vi "10-Tap 8-Bit Camera with DRAM (Host).vi"() -> ()   [LabVIEW 2014]
doc: "This is the host VI for the 10-Tap 8-Bit Camera with DRAM example. This example demonstrates how to acquire images from a 10-tap, 8-bit, extended configuration, Camera Link camera and display the images on the host. This example supports area scan and line scan cameras for both continuous and finite acquisitions.\n\nThis example also demonstrates the use of DRAM as a frame buffer for very high speed acquisitions. Data packing and flow-control are also employed to maximize use of the available DRAM and FIFOs in terms of both memory space and performance.\n\nAdditionally, the example demonstrates the serial server, which allows third-party camera configuration utilities to communicate with the camera using the Camera Link serial interface while this VI is running."
uses:
  <vilib>/userdefined/High Color/nirio_resource_hc.ctl
  <vilib>/DAQmx/write.llb/DAQmx Write (Analog DBL 1Chan 1Samp).vi
  <vilib>/FPGAPlugInAG/PCIe-1473R/niLvFpga_Open_PCIe-1473R.vi
  <vilib>/rvi/interface/common/dynamic/niFpgaDynamicAddResources.vi
  <vilib>/FPGAPlugInAG/Dynamic/niLvFpga_Reset_Dynamic.vi
  <vilib>/Utility/error.llb/Error Cluster From Error Code.vi
  <vilib>/rvi/errors/niLvFpgaAdjustHostInterfaceError.vi
  <vilib>/FPGAPlugInAG/Dynamic/niLvFpga_Run_Dynamic.vi
  <vilib>/rvi/interface/common/niFpgaWaitOnOcc.vi
  <vilib>/FPGAPlugInAG/Dynamic/niLvFpga_Close_Dynamic.vi
  <vilib>/rvi/interface/nirviOpenFPGA/nirviOpenFPGA.xnode
  FPGA Bitfiles/10-Tap8-bitCamer_FPGATarget_10-Tap8-bitCamer_C490DC32.lvbitx
  10-Tap 8-Bit Camera with DRAM(FPGA).vi
  <vilib>/rvi/interface/nirviMethod/nirviMethod.xnode
  <vilib>/rvi/interface/nirviReadWriteControl/nirviReadWriteControl.xnode
  <vilib>/rvi/interface/nirviCloseFPGA/nirviCloseFPGA.xnode
  <vilib>/rvi/interface/Simulation/niFpgaSimulationCallBeginRW.vi
  <vilib>/rvi/errors/niLvFpgaMergeErrorWithErrorCode.vi
  NiFpgaLv.dll
  <vilib>/FPGAPlugInAG/Dynamic/niLvFpga_ConfigureFifo_Dynamic.vi
  <vilib>/FPGAPlugInAG/Dynamic/niLvFpga_StartFifo_Dynamic.vi
  <vilib>/FPGAPlugInAG/Dynamic/niLvFpga_ReadFifo_Dynamic.vi
  <vilib>/vision/NI_Vision_Development_Module.lvlib
panel:
  out "YofFishHead":sgl
  out "XofFishHead":dbl
  in  "Ly":sgl=30.0
  in  "Lx":dbl=50.0
  out "TimeDelay":dbl
  out "RegionSelected":T1(plugin-control)
  in  "Threshold":u8=96
  out "Objects":T2(array[cluster]) {"Aspect Ratio" format="%.2f"; "Orientation" format="%.2f"; "Area" format="%.2f"; "Object Center"."Y" format="%.2f"; "Object Center"."X" format="%.2f"}
  in  "Machine Vision Settings":T3={"Objects"=0, "Threshold"=128, "Reject Border"=FALSE, "Fill Holes"=FALSE, "Min Object Size"=TRUE, "Min Size"=10000, "Max Object Size"=FALSE, "Max Size"=100, "Show Search Area"=FALSE, "Show Center"=TRUE, "Show Bounding Box"=TRUE} {"Objects" items=["Bright Objects", "Dark Objects"]; "Threshold" min=1 max=999999999 step=1; "Max Size" min=1 max=999999999 step=1; "Min Size" min=1 max=999999999 step=1}
  in  "长度2_LeftToRight":i32=300
  in  "索引2_LeftEdge":i32=250
  in  "长度1_UpToLow":i32=400
  in  "索引1_UpEdge":i32=290
  out "image":u8[][](array[numeric])
  in  "SpeedFactor":dbl=1.0
  in  "Offset":dbl=150.0
  in  "Y_Target":dbl=384.0
  in  "X_Target":dbl=520.0
  in  "Y_LowEdge_ofCenter":fxp<+,32,16>=440.0 format="%#_21g"
  in  "X_RightEdge_ofCenter":fxp<+,32,16>=600.0 format="%#_21g"
  in  "Y_HighEdge_ofCenter":fxp<+,32,16>=270.0 format="%#_21g"
  in  "X_LeftEdge_ofCenter":fxp<+,32,16>=440.0 format="%#_21g"
  out "Y_edge":u16[](array[numeric])
  out "X_edge":u16[](array[numeric])
  out "Centroid":fxp<+,32,16>[](array[numeric])
  in  "DMA Buffer Size\n(In Images)":u32=64 caption="DMA Buffer Size"
  in  "Signal Mapping":T4(ring)=enum."Basler 10-tap"
  out "Acq In Progress":bool
  in  "Line Scan":bool
  in  "Frames To Acquire":u32 caption="Frames To Acquire\n(0 = infinite)"
  in  "Cancel":bool
  out "Acq'd Frame Width":u32
  in  "Stopped":bool
  in  "RIO Device":T5="Horizontal"
  out "DMA Write Timeout":bool
  in  "Start Serial Server":bool=TRUE
  out "Frames Acq'd":u32
  out "Acq'd Frame Height":u32
  out "Image":T1(plugin-control)
  in  "Acquire":bool
  in  "Stop":bool
  in  "Image Height":u32=768 max=65535
  in  "Image Width":u32=1040 max=65535 step=40
  out "Initialized":bool
  # "对鱼的不同方位进行不同的微调。"
  # "右边四个参数是一个\n长方形框的四个边，\n只有当FPGA计算出来\n的中心在这个框内的\n时候才会使用PC进行\n处理。"
  # "右边四个参数也是\n一个长方形的框，\n他是PC进行处理的\n范围，它的大小直\n接影响PC处理的速\n度。"
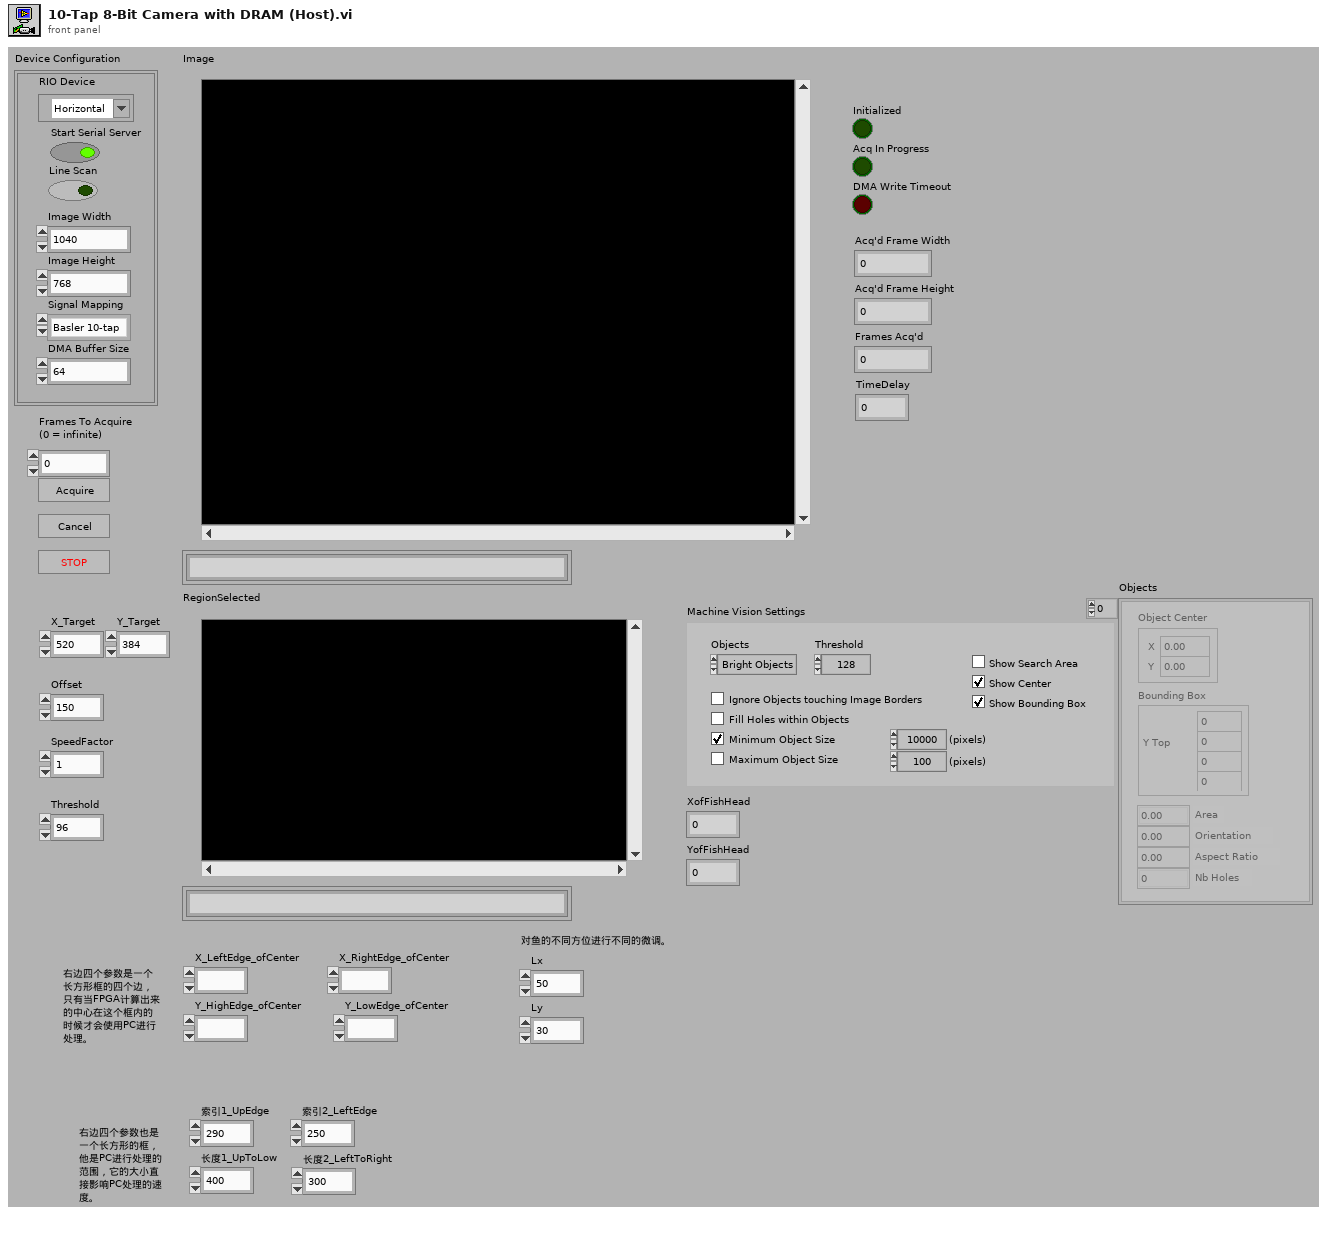
[diagram p1: front panel]
types:
  T1 = typedef "IMAQ Image.ctl" = refnum<image>
  T2 = cluster{"Object Center":cluster{"X":sgl, "Y":sgl}, "Bounding Box":cluster{"X Left":i32, "Y Top":i32, "X Right":i32, "Y Bottom":i32}, "Area":sgl, "Orientation":sgl, "Aspect Ratio":sgl, "Nb Holes":i32}[]
  T3 = cluster{"Objects":u16, "Threshold":i32, "Reject Border":bool, "Fill Holes":bool, "Min Object Size":bool, "Min Size":i32, "Max Object Size":bool, "Max Size":i32, "Show Search Area":bool, "Show Center":bool, "Show Bounding Box":bool}
  T4 = enum8{"Standard", "Basler 10-tap", "Vosskühler 10-tap"}
  T5 = typedef "nirio_resource_hc.ctl" = tag
  T6 = typedef "Image Type" = u32
  T7 = enum16{"big-endian, network order", "native, host order", "little-endian"}
  T8 = enum32{"AutoM", "Close", "Dilate", "Erode", "Gradient", "Gradient out", "Gradient in", "Hit miss", "Open", "PClose", "POpen", "Thick", "Thin"}
  T9 = cluster{"Object Center":cluster{"X":sgl, "Y":sgl}, "Bounding Box":cluster{"X Left":i32, "Y Top":i32, "X Right":i32, "Y Bottom":i32}, "Area":sgl, "Orientation":sgl, "Aspect Ratio":sgl, "Nb Holes":i32}
  T10 = cluster{"X Left":i32, "Y Top":i32, "X Right":i32, "Y Bottom":i32}
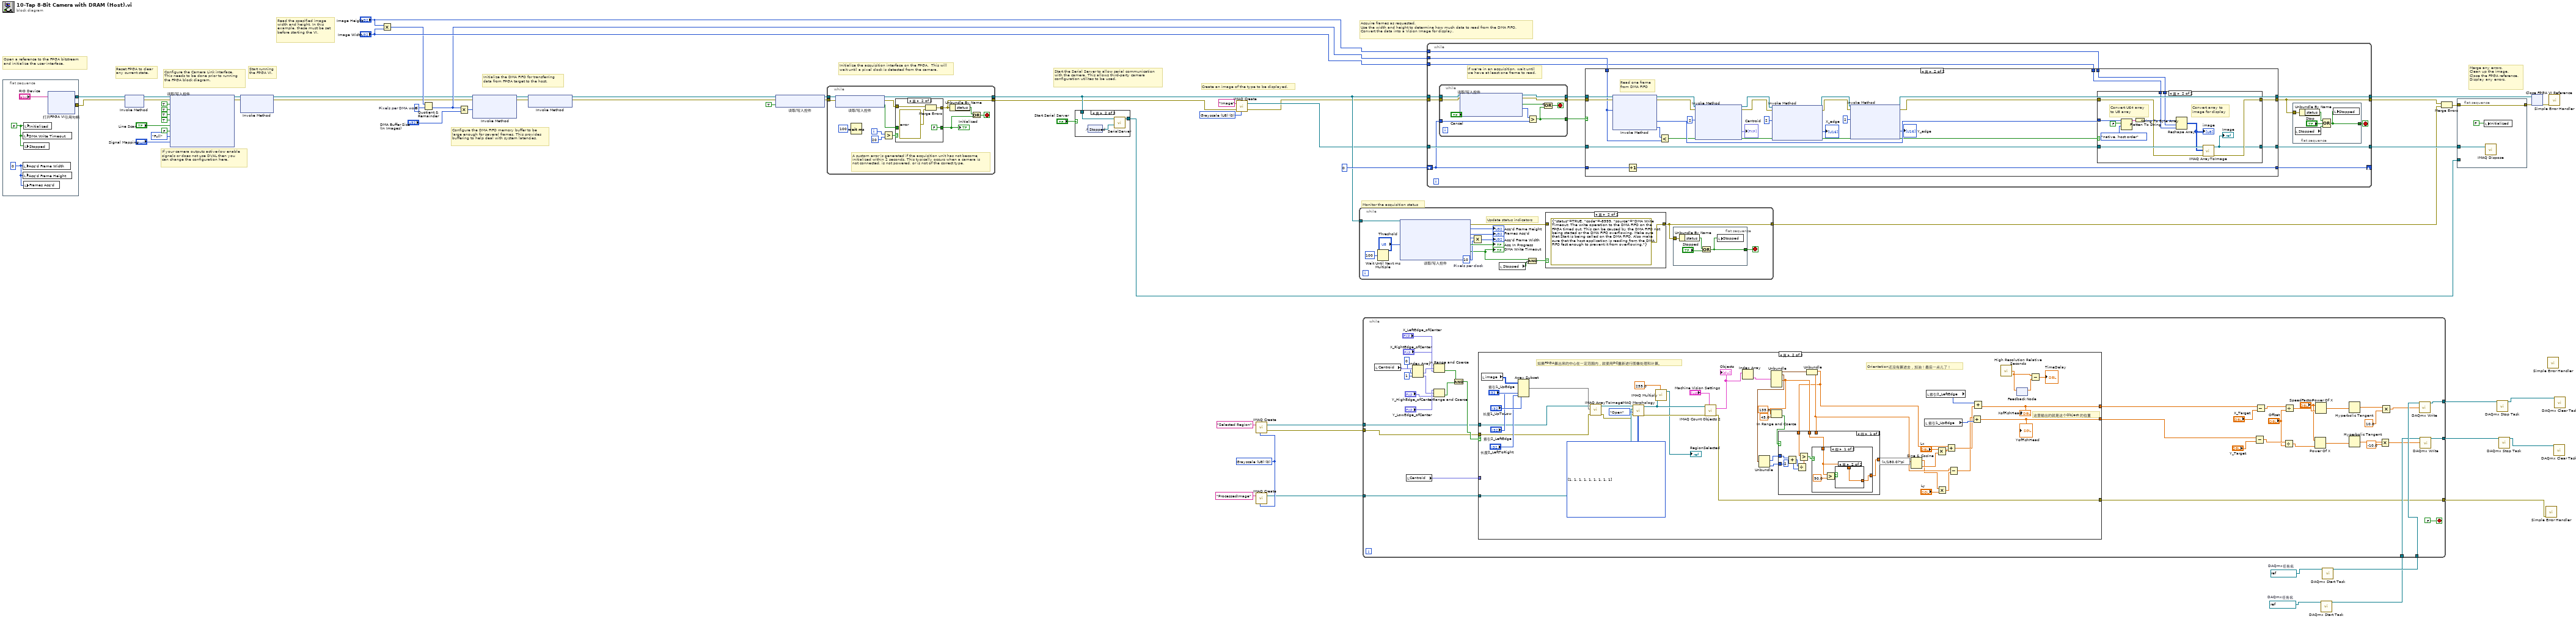
[diagram p0: block diagram]
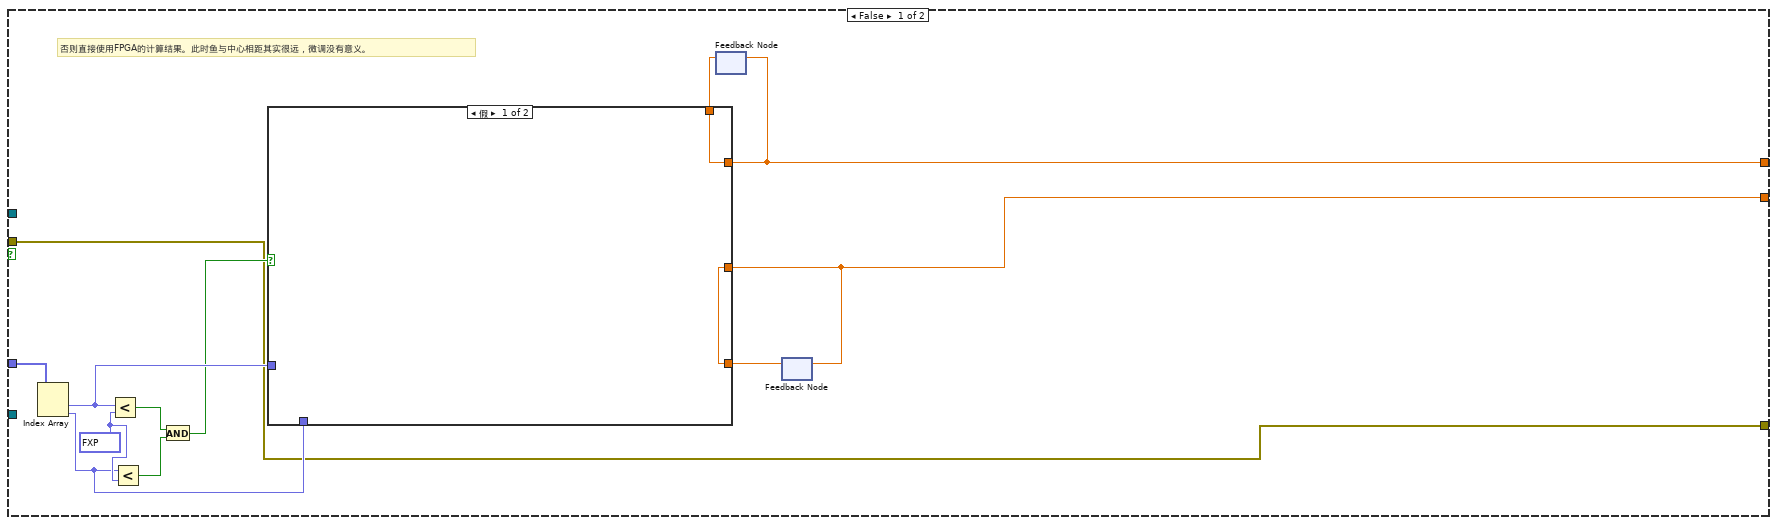
[diagram p2: hidden frame]
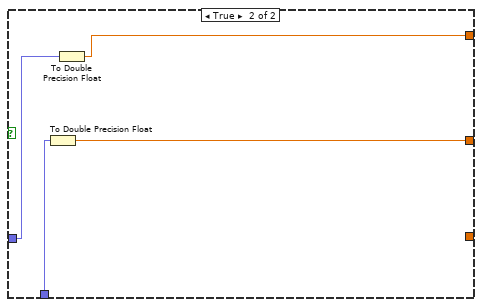
[diagram p3: hidden frame]
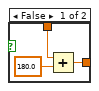
[diagram p4: hidden frame]
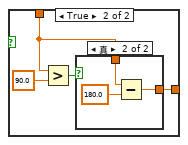
[diagram p5: hidden frame]
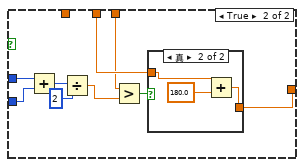
[diagram p7: hidden frame]
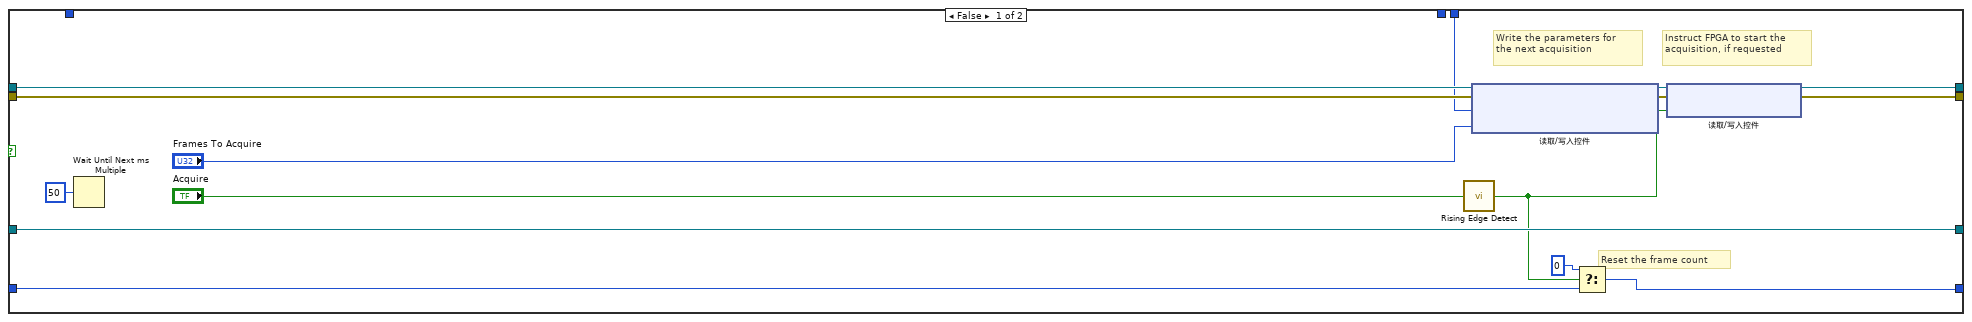
[diagram p11: hidden frame]
diagram:
  w4 = T6 0 items=["Grayscale (U8)", "Grayscale (I16)", "Grayscale (SGL)", "Complex (CSG)", "RGB (U32)", "HSL (U32)", "RGB (U64)", "Grayscale (U16)"] ("Image Type")
  w12 = refnum<k21> "Stage_Y"  # DAQmx任务名
  w15 = refnum<k21> "Stage_X"  # DAQmx任务名
  w21 = u32 8  # Pixels per DMA word
  w57 = T6 0 items=["Grayscale (U8)", "Grayscale (I16)", "Grayscale (SGL)", "Complex (CSG)", "RGB (U32)", "HSL (U32)", "RGB (U64)", "Grayscale (U16)"] ("Image Type")
  # "If your camera outputs active-low enable\nsignals or does not use DVAL then you \ncan change the configuration here."
  # "Configure the DMA FIFO memory buffer to be\nlarge enough for several frames. This provides\nbuffering to help deal with system latencies."
  # "Start running\nthe FPGA VI."
  # "Reset FPGA to clear\nany current state."
  # "Read the specified image\nwidth and height. In this\nexample, these must be set\nbefore starting the VI."
  # "Merge any errors.\nClean up the image.\nClose the FPGA reference.\nDisplay any errors."
  # "Acquire frames as requested.\nUse the width and height to determine how much data to read from the DMA FIFO.\nConvert the data into a Vision Image for display."
  # "Monitor the acquisition status"
  # "Start the Serial Server to allow serial communication\nwith the camera. This allows third-party camera\nconfiguration utilites to be used."
  # "Create an image of the type to be displayed."
  # "Initialize the acquisition interface on the FPGA.  This will\nwait until a pixel clock is detected from the camera."
  # "Initialize the DMA FIFO for transferring\ndata from FPGA target to the host."
  # "Configure the Camera Link interface.\nThis needs to be done prior to running\nthe FPGA block diagram."
  # "Open a reference to the FPGA bitstream\nand initialize the user interface."
  n1 = flat-sequence {
    tunnel: [w63] -> w48
    tunnel: [w62] -> w61
    frame #0 {
      w66 = u32 0 ("Num Lines Acq'd")
      w65 = FALSE ("stop")
      n2 = local write "DMA Write Timeout"(w65) -> ()
      n3 = local write "Acq'd Frame Width"(w66) -> ()
      n4 = local write "Acq'd Frame Height"(w66) -> ()
      n5 = local write "Stopped"(w65) -> ()
      n6 = local write "Frames Acq'd"(w66) -> ()
      n7 = local write "Initialized"(w65) -> ()
      n8 = xnode "打开FPGA VI引用句柄"("资源名称"="RIO Device") -> ("FPGA VI引用输出"=w63:refnum<k20>, "错误输出"=w62:errorcluster)  [unwired: 1 in]
    }
  }
  n9 = xnode "Invoke Method"("FPGA VI引用输入"=w48, "错误输入"=w61) -> ("FPGA VI引用输出"=w38:refnum<k20>, "错误输出"=w41:errorcluster)
  n10 = xnode "读取/写入控件"("FPGA VI引用输入"=w38, "错误输入"=w41, "CL Config.FVAL Active High"=TRUE ("IO Module Config.CL FVAL Active High"), "CL Config.LVAL Active High"=TRUE ("IO Module Config.CL LVAL Active High"), "CL Config.DVAL Active High"=TRUE ("IO Module Config.CL DVAL Active High"), "CL Config.Spare Active High"=TRUE ("IO Module Config.CL Spare Active High"), "CL Config.Line Scan"="Line Scan", "Acq Control.Ignore DVAL"=FALSE ("CL Config.Line Scan"), "CL Config.Configuration"=enum8{"Base", "Medium", "Full"}."Full", "CL Config.Signal Mapping"="Signal Mapping") -> ("FPGA VI引用输出"=w42:refnum<k20>, "错误输出"=w40:errorcluster)
  n11 = xnode "Invoke Method"("FPGA VI引用输入"=w42, "错误输入"=w40) -> ("FPGA VI引用输出"=w18:refnum<k20>, "错误输出"=w17:errorcluster)  [unwired: 1 in]
  n12 = Multiply(x="Image Height", y="Image Width") -> (x*y=w20:u32)
  n13 = Quotient & Remainder(x=w20, y=w21) -> (floor(x/y)=w19:u32)  [unwired: 1 out]
  n14 = Multiply(x=w19, y="DMA Buffer Size\n(In Images)") -> (x*y=w32:u32)
  n15 = xnode "Invoke Method"("FPGA VI引用输入"=w18, "错误输入"=w17, "请求的深度"=w32) -> ("FPGA VI引用输出"=w16:refnum<k20>, "错误输出"=w47:errorcluster)  [unwired: 1 out]
  n16 = xnode "Invoke Method"("FPGA VI引用输入"=w16, "错误输入"=w47) -> ("FPGA VI引用输出"=w33:refnum<k20>, "错误输出"=w46:errorcluster)
  n17 = xnode "读取/写入控件"("FPGA VI引用输入"=w33, "错误输入"=w46, "Acq Control.Initialize"=TRUE ("Arm Acquisition")) -> ("FPGA VI引用输出"=w60:refnum<k20>, "错误输出"=w59:errorcluster)
  n18 = while {
    tunnel: w60 -> [w74]
    tunnel: w59 -> [w73]
    tunnel: [w72] -> w29
    tunnel: [w76] -> w28
    i -> [w68]
    stop <- w79 stop-if-true
    # "A custom error is generated if the acquisition unit has not become\ninitialized within 2 seconds. This typically occurs when a camera is\nnot connected, is not powered, or is not of the correct type."
    n19 = xnode "读取/写入控件"("FPGA VI引用输入"=w74, "错误输入"=w73) -> ("FPGA VI引用输出"=w72:refnum<k20>, "错误输出"=w71:errorcluster, "Acq Status.Initialized"=w70:bool)
    n20 = Wait (ms)(milliseconds to wait=u32 100) -> ()  [unwired: 1 out]
    n21 = Greater?(x=w68, y=20) -> (0:w69:bool)
    n22 = case shown="真" w69 {
      tunnel: [w81 FALSE] -> w75
      tunnel: w70 -> [w81 _]
      tunnel: w71 -> [w80 w83]
      tunnel: [w80 w85] -> w76
      frame False {
      }
      frame True {
        n23 = Merge Errors(w83, errorcluster {"status"=TRUE, "code"=-8999, "source"="Acquisition Initialization: This error typically occurs when a camera is not properly connected, is not powered, or is not of the correct type."} ("error in")) -> (w85:errorcluster)
      }
    }
    "Initialized" <- w75
    n24 = Unbundle By Name(w76) -> ("status"=w78:bool)
    n25 = Or(x=w78, y=w75) -> (x .or. y?=w79:bool)
  }
  n26 = case shown="真" "Start Serial Server" {
    tunnel: [_ w86] -> w49
    tunnel: w29 -> [_ w87]
    frame False {
    }
    frame True {
      n27 = control-ref of="Stopped"() -> (w88:refnum<vi>)
      n28 = call "SerialServer.vi"("Stop Refnum"=w88, "FPGA VI Reference In"=w87) -> ("FPGA VI Reference Out"=w86:refnum<k20>)  [unwired: 5 in]
    }
  }
  n29 = call "IMAQ Create"("Image Name"="Image", "Image Type"=w57, "error in (no error)"=w28) -> ("New Image"=w25:T1, "error out"=w24:errorcluster)  [unwired: 2 in]
  n30 = call "IMAQ Create"("Image Name"="Selected Region", "Image Type"=w4) -> ("New Image"=w6:T1, "error out"=w5:errorcluster)  [unwired: 3 in]
  n31 = call "IMAQ Create"("Image Name"="ProcessedImage", "Image Type"=w4) -> ("New Image"=w2:T1)  [unwired: 3 in, 1 out]
  n32 = while {
    tunnel: w29 -> [w100]
    tunnel: [w103] -> w43
    stop <- w102 stop-if-true
    w93 = u32 10  # Pixels per clock
    # "Update status indicators"
    n33 = Wait Until Next ms Multiple(millisecond multiple=u32 100) -> ()  [unwired: 1 out]
    n34 = xnode "读取/写入控件"("FPGA VI引用输入"=w100, "Threshold"="Threshold") -> ("错误输出"=w99:errorcluster, "Acq Status.Lines Per Frame"=→"Acq'd Frame Height":u32, "Acq Status.Frames Acq'd"=→"Frames Acq'd":u32, "Acq Status.Clocks Per Line"=w94:u32, "Acq Status.Acq In Progress"=→"Acq In Progress":bool, "Acq Status.DMA Write Timeout"=w91:bool)  [unwired: 1 in, 1 out]
    "DMA Write Timeout" <- w91
    n35 = Multiply(x=w94, y=w93) -> (x*y=→"Acq'd Frame Width":u32)
    n36 = local read "Stopped"() -> (w90:bool)
    n37 = Compound Arithmetic op=AND(w91, invert w90) -> (w92:bool)
    n38 = case shown="真" w92 {
      tunnel: w99 -> [w108 _]
      tunnel: [w108 errorcluster {"status"=TRUE, "code"=-8999, "source"="DMA Write Timeout: The write operation to the DMA FIFO on the FPGA timed out. This can be caused by the DMA FIFO not being started or the DMA FIFO overflowing. Make sure that Start is being called on the DMA FIFO. Also make sure that the host application is reading from the DMA FIFO fast enough to prevent it from overflowing."} ("error out")] -> w103
      frame False {
      }
      frame True {
      }
    }
    n39 = flat-sequence {
      tunnel: w103 -> [w107]
      tunnel: [w105] -> w102
      frame #0 {
        n40 = Unbundle By Name(w107) -> ("status"=w106:bool)
        n41 = Or(x=w106, y="Stopped") -> (x .or. y?=w105:bool)
        n42 = local write "Stopped"(w105) -> ()
      }
    }
  }
  n43 = while {
    tunnel: w29 -> [w116]
    tunnel: w24 -> [w115]
    tunnel: w19 -> [w124]
    tunnel: "Image Height" -> [w123]
    tunnel: "Image Width" -> [w122]
    tunnel: w25 -> [w121]
    tunnel: [w119] -> w44
    tunnel: [w120] -> w56
    tunnel: [w117] -> w51
    shift-right: [w111] -> _
    shift-left: u32 0 -> [w110]
    stop <- w118 stop-if-true
    # "If we're in an acquisition, wait until\nwe have at least one frame to read."
    n44 = while {
      tunnel: w116 -> [w131]
      tunnel: w115 -> [w130]
      tunnel: [w128] -> w114
      tunnel: [w129] -> w113
      tunnel: w110 -> [w134]
      tunnel: [w132] -> w112
      stop <- w133 stop-if-true
      n45 = xnode "读取/写入控件"("FPGA VI引用输入"=w131, "错误输入"=w130, "Acq Control.Cancel Acq"="Cancel") -> ("FPGA VI引用输出"=w129:refnum<k20>, "错误输出"=w128:errorcluster, "Acq Status.Acq In Progress"=w127:bool, "Acq Status.Frames Acq'd"=w126:u32)
      n46 = Greater?(x=w126, y=w134) -> (0:w132:bool)
      n47 = Compound Arithmetic op=OR(invert w127, w132) -> (w133:bool)
    }
    n48 = case shown="真" w112 {
      tunnel: w113 -> [w150 w176]
      tunnel: w114 -> [w149 w175]
      tunnel: w124 -> [_ w169]
      tunnel: w123 -> [w143 w181]
      tunnel: w122 -> [_ w180]
      tunnel: w121 -> [w154 w179]
      tunnel: [w145 w178] -> w119
      tunnel: [w148 w162] -> w120
      tunnel: [w154 w177] -> w117
      tunnel: w110 -> [w151 w174]
      tunnel: [w153 w173] -> w111
      frame False {
        # "Reset the frame count"
        # "Instruct FPGA to start the\nacquisition, if requested"
        # "Write the parameters for\nthe next acquisition"
        n49 = Wait Until Next ms Multiple(millisecond multiple=u32 50) -> ()  [unwired: 1 out]
        n50 = call "Rising Edge Detect.vi"("Input"="Acquire") -> ("Pulse"=w140:bool)  [unwired: 4 in]
        n51 = xnode "读取/写入控件"("FPGA VI引用输入"=w150, "错误输入"=w149, "Acq Control.Line Scan Height"=w143, "Acq Control.Frames To Acq"="Frames To Acquire") -> ("FPGA VI引用输出"=w147:refnum<k20>, "错误输出"=w146:errorcluster)
        n52 = Select(t=u32 0, s=w140, f=w151) -> (s? t:f=w153:u32)
        n53 = xnode "读取/写入控件"("FPGA VI引用输入"=w147, "错误输入"=w146, "Acq Control.Acquire"=w140) -> ("FPGA VI引用输出"=w148:refnum<k20>, "错误输出"=w145:errorcluster)
      }
      frame True {
        # "Read one frame\nfrom DMA FIFO"
        n54 = xnode "Invoke Method"("FPGA VI引用输入"=w176, "错误输入"=w175, "元素数量"=w169) -> ("FPGA VI引用输出"=w168:refnum<k20>, "错误输出"=w167:errorcluster, "数据"=w172:u64[], "剩余元素"=w170:u32)  [unwired: 1 in]
        n55 = Increment(x=w174) -> (x+1=w173:u32)
        n56 = Less?(x=w170, y=w169) -> (x < y?=w171:bool)
        n57 = xnode "Invoke Method"("FPGA VI引用输入"=w168, "错误输入"=w167, "元素数量"=u32 2) -> ("FPGA VI引用输出"=w165:refnum<k20>, "错误输出"=w164:errorcluster, "数据"=→"Centroid":fxp<+,32,16>[])  [unwired: 1 in, 1 out]
        n58 = xnode "Invoke Method"("FPGA VI引用输入"=w165, "错误输入"=w164, "元素数量"=u32 2) -> ("FPGA VI引用输出"=w163:refnum<k20>, "错误输出"=w161:errorcluster, "数据"=→"X_edge":u16[])  [unwired: 1 in, 1 out]
        n59 = xnode "Invoke Method"("FPGA VI引用输入"=w163, "错误输入"=w161, "元素数量"=u32 2) -> ("FPGA VI引用输出"=w162:refnum<k20>, "错误输出"=w160:errorcluster, "数据"=→"Y_edge":u16[])  [unwired: 1 in, 1 out]
        n60 = case shown="真" w171 {
          tunnel: w181 -> [_ w195]
          tunnel: w180 -> [_ w194]
          tunnel: w179 -> [w183 w193]
          tunnel: w160 -> [w182 w192]
          tunnel: [w182 w191] -> w178
          tunnel: [w183 w190] -> w177
          tunnel: w172 -> [_ w187]
          frame False {
            # "Do not display the image if we're falling behind in the acquisition."
          }
          frame True {
            # "Convert U64 array\nto U8 array"
            # "Convert array to\nimage for display"
            n61 = Flatten To String(anything=w187, prepend array or string size? (T)=FALSE, byte order (0:big-endian, network order)=T7."native, host order") -> (data string=w185:string)  [unwired: 1 in, 2 out]
            n62 = String To Byte Array(string=w185) -> (unsigned byte array=w184:u8[])
            n63 = Reshape Array(w184, w195, w194) -> (w189:u8[][])
            "image" <- w189
            n64 = call "IMAQ ArrayToImage"("error in (no error)"=w192, "Image Pixels (U8)"=w189, "Image"=w193) -> ("error out"=w191:errorcluster, "Image Out"=w190:T1)  [unwired: 7 in]
            "Image" <- w190
          }
        }
      }
    }
    n65 = flat-sequence {
      tunnel: w119 -> [w137]
      tunnel: [w136] -> w118
      frame #0 {
        n66 = local read "Stopped"() -> (w135:bool)
        n67 = Unbundle By Name(w137) -> ("status"=w138:bool)
        n68 = Compound Arithmetic op=OR(w138, "Stop", w135) -> (w136:bool)
        n69 = local write "Stopped"(w136) -> ()
      }
    }
  }
  n70 = call <vilib>:"DAQmx Start Task.vi"("task/channels in"=w12) -> ("task out"=w13:refnum<k21>)  [unwired: 13 in, 1 out]
  n71 = call <vilib>:"DAQmx Start Task.vi"("task/channels in"=w15) -> ("task out"=w14:refnum<k21>)  [unwired: 13 in, 1 out]
  n72 = while {
    tunnel: w14 -> [w228]
    tunnel: w13 -> [w227]
    tunnel: [w226] -> w11
    tunnel: [w225] -> w10
    tunnel: w6 -> [w206]
    tunnel: w5 -> [w205]
    tunnel: w2 -> [w204]
    tunnel: [w202] -> w1
    stop <- FALSE stop-if-true
    n73 = local read "Centroid"() -> (w235:fxp<+,32,16>[])
    n74 = local read "Centroid"() -> (w224:fxp<+,32,16>[])
    n75 = Index Array(array=w235, index #1=0 ("索引"), index #2=1 ("索引")) -> (element #1=w234:fxp<+,32,16>, element #2=w231:fxp<+,32,16>)
    n76 = In Range and Coerce(upper limit="Y_LowEdge_ofCenter", x=w231, lower limit="Y_HighEdge_ofCenter") -> (In Range?=w229:bool)  [unwired: 1 out]
    n77 = In Range and Coerce(upper limit="X_RightEdge_ofCenter", x=w234, lower limit="X_LeftEdge_ofCenter") -> (In Range?=w230:bool)  [unwired: 1 out]
    n78 = And(x=w230, y=w229) -> (x .and. y?=w207:bool)
    n79 = case shown="真" w207 {
      tunnel: w224 -> [w247 _]
      tunnel: [w240 w283] -> w221
      tunnel: [w238 w281] -> w219
      tunnel: w206 -> [_ w295]
      tunnel: w205 -> [w236 w294]
      tunnel: w204 -> [_ w291]
      tunnel: [w236 w284] -> w202
      frame False {
        w246 = fxp<+,32,16> 10000.0 ("y")
        # "否则直接使用FPGA的计算结果。此时鱼与中心相距其实很远，微调没有意义。"
        n80 = Index Array(array=w247) -> (element #1=w243:fxp<+,32,16>, element #2=w242:fxp<+,32,16>)  [unwired: 2 in]
        n81 = Less?(x=w243, y=w246) -> (x < y?=w245:bool)
        n82 = Less?(x=w242, y=w246) -> (x < y?=w244:bool)
        n83 = And(x=w245, y=w244) -> (x .and. y?=w241:bool)
        n84 = feedback #1() -> (w239:dbl)  [unwired: 1 in]
        n85 = feedback #2() -> (w237:dbl)  [unwired: 1 in]
        n86 = case shown="假" w241 {
          tunnel: w243 -> [_ w253]
          tunnel: w242 -> [_ w252]
          tunnel: [w249 w251] -> w240
          tunnel: [w248 w250] -> w238
          tunnel: w239 -> [w249 _]
          tunnel: w237 -> [w248 _]
          frame False {
          }
          frame True {
            n87 = To Double Precision Float(number=w252) -> (double precision float=w250:dbl)
            n88 = To Double Precision Float(number=w253) -> (double precision float=w251:dbl)
          }
        }
        n89 = feedback-in #1(w240) -> ()
        n90 = feedback-in #2(w238) -> ()
      }
      frame True {
        # "如果FPGA算出来的中心在一定范围内，就使用PC重新进行图像处理和计算。"
        # "Orientation还没有算进去，加油！最后一点儿了！"
        # "这里输出的就是这个Object 的位置"
        n91 = local read "image"() -> (w301:u8[][])
        n92 = Array Subset(array=w301, index (row)="索引1_UpEdge", length (row)="长度1_UpToLow", index (col)="索引2_LeftEdge", length (col)="长度2_LeftToRight") -> (w296:u8[][])
        n93 = call "IMAQ ArrayToImage"("error in (no error)"=w294, "Image Pixels (U8)"=w296, "Image"=w295) -> ("error out"=w290:errorcluster, "Image Out"=w292:T1)  [unwired: 7 in]
        n94 = call "IMAQ Morphology"("Structuring Element"=i32[][] [[1, 1, 1], [1, 1, 1], [1, 1, 1]], "error in (no error)"=w290, "Operation"=T8."Open", "Image Dst"=w291, "Image Src"=w292) -> ("error out"=w289:errorcluster, "Image Dst Out"=w279:T1)  [unwired: 5 in]
        n95 = call "IMAQ Multiply"("Image Src A"=w279, "Constant"=255.0) -> ("Image Dst Out"=→"RegionSelected":T1)  [unwired: 5 in, 1 out]
        n96 = call "IMAQ Count Objects 2"("Settings"="Machine Vision Settings", "error in (no error)"=w289, "Image"=w279) -> ("error out"=w284:errorcluster, "Objects"=w276:T2)  [unwired: 4 in, 3 out]
        "Objects" <- w276
        n97 = Index Array(array=w276) -> (element=w286:T9)  [unwired: 1 in]
        n98 = Unbundle(w286) -> ("Object Center"=w285:cluster{"X":sgl, "Y":sgl}, "Bounding Box"=w272:T10, "Orientation"=w258:sgl)  [unwired: 3 out]
        n99 = Unbundle(w272) -> ("Y Top"=w271:i32, "Y Bottom"=w270:i32)  [unwired: 2 out]
        n100 = In Range and Coerce(upper limit=sgl 135.0 ("上限"), x=w258, lower limit=sgl 45.0 ("下限")) -> (In Range?=w255:bool)  [unwired: 1 out]
        n101 = Unbundle(w285) -> ("X"=w254:sgl, "Y"=w263:sgl)
        n102 = case shown="假" w255 {
          tunnel: w271 -> [w310 w332]
          tunnel: w270 -> [w309 w331]
          tunnel: w258 -> [w303 w329]
          tunnel: [w302 w328] -> w267
          tunnel: w263 -> [_ w327]
          tunnel: w254 -> [w307 _]
          frame False {
            n103 = Add(x=w310, y=w309) -> (x+y=w308:i32)
            n104 = Divide(x=w308, y=2) -> (x/y=w305:dbl)
            n105 = Greater?(x=w307, y=w305) -> (0:w306:bool)
            n106 = case shown="假" w306 {
              tunnel: w303 -> [w312 w320]
              tunnel: [w311 w319] -> w302
              frame False {
                n107 = Greater?(x=w312, y=90.0) -> (0:w313:bool)
                n108 = case shown="真" w313 {
                  tunnel: w312 -> [w316 w318]
                  tunnel: [w315 w318] -> w311
                  frame False {
                    n109 = Add(x=w316, y=180.0) -> (x+y=w315:dbl)
                  }
                  frame True {
                  }
                }
              }
              frame True {
                n110 = Greater?(x=w320, y=90.0) -> (0:w321:bool)
                n111 = case shown="真" w321 {
                  tunnel: w320 -> [w323 w325]
                  tunnel: [w323 w324] -> w319
                  frame False {
                  }
                  frame True {
                    n112 = Subtract(x=w325, y=180.0) -> (x-y=w324:dbl)
                  }
                }
              }
            }
          }
          frame True {
            n113 = Add(x=w332, y=w331) -> (x+y=w335:i32)
            n114 = Divide(x=w335, y=2) -> (x/y=w333:dbl)
            n115 = Greater?(x=w327, y=w333) -> (0:w330:bool)
            n116 = case shown="真" w330 {
              tunnel: w329 -> [w336 w339]
              tunnel: [w336 w337] -> w328
              frame False {
              }
              frame True {
                n117 = Add(x=w339, y=sgl 180.0) -> (x+y=w337:sgl)
              }
            }
          }
        }
        n118 = expression code="(x/180.0)*pi" ("degrees to radians")(w267) -> (w266:dbl)
        n119 = Sine & Cosine(0:w266) -> (1:w261:dbl, 2:w265:dbl)
        n120 = local read "索引1_UpEdge"() -> (w280:i32)
        n121 = local read "索引2_LeftEdge"() -> (w282:i32)
        n122 = Multiply(x="Lx", y=w265) -> (x*y=w269:dbl)
        n123 = Multiply(x=w261, y="Ly") -> (x*y=w262:dbl)
        n124 = Add(x=w254, y=w269) -> (x+y=w264:dbl)
        n125 = Subtract(x=w263, y=w262) -> (x-y=w259:dbl)
        n126 = Add(x=w259, y=w280) -> (x+y=w281:dbl)
        "YofFishHead" <- w281
        n127 = Add(x=w282, y=w264) -> (x+y=w283:dbl)
        "XofFishHead" <- w283
        n128 = call <vilib>:"High Resolution Relative Seconds.vi"() -> ("relative seconds"=w275:dbl)
        n129 = feedback-in #3(w275) -> ()
        n130 = feedback #3() -> (w274:dbl)  [unwired: 1 in]
        n131 = Subtract(x=w275, y=w274) -> (x-y=→"TimeDelay":dbl)
      }
    }
    n132 = Subtract(x=w219, y="Y_Target") -> (x-y=w216:dbl)
    n133 = Subtract(x=w221, y="X_Target") -> (x-y=w217:dbl)
    n134 = Divide(x=w216, y="Offset") -> (x/y=w213:dbl)
    n135 = Divide(x=w217, y="Offset") -> (x/y=w214:dbl)
    n136 = Power Of X(1:w213, 2:"SpeedFactor") -> (0:w210:dbl)
    n137 = Power Of X(1:w214, 2:"SpeedFactor") -> (0:w211:dbl)
    n138 = Hyperbolic Tangent(1:w211) -> (0:w209:dbl)
    n139 = Hyperbolic Tangent(1:w210) -> (0:w208:dbl)
    n140 = Multiply(x=w208, y=-10.0) -> (x*y=w222:dbl)
    n141 = Multiply(x=w209, y=10.0) -> (x*y=w223:dbl)
    n142 = call-poly <vilib>:"DAQmx Write.vi"("task/channels in"=w228, "data"=w223) -> ("task out"=w226:refnum<k21>)  [unwired: 11 in, 2 out]
    n143 = call-poly <vilib>:"DAQmx Write.vi"("task/channels in"=w227, "data"=w222) -> ("task out"=w225:refnum<k21>)  [unwired: 11 in, 2 out]
  }
  n144 = Merge Errors(w44, w43) -> (w45:errorcluster)
  n145 = flat-sequence {
    tunnel: w45 -> [w341]
    tunnel: [w341] -> w53
    tunnel: w51 -> [w342]
    tunnel: w49 -> [_]
    frame #0 {
      n146 = local write "Initialized"(FALSE ("Module Enabled")) -> ()
      n147 = call "IMAQ Dispose"("Image"=w342) -> ()  [unwired: 5 in, 1 out]
    }
  }
  n148 = call <vilib>:"DAQmx Stop Task.vi"("task/channels in"=w11) -> ("task out"=w9:refnum<k21>)  [unwired: 13 in, 1 out]
  n149 = call <vilib>:"DAQmx Stop Task.vi"("task/channels in"=w10) -> ("task out"=w8:refnum<k21>)  [unwired: 13 in, 1 out]
  n150 = xnode "Close FPGA VI Reference"("FPGA VI引用输入"=w56, "错误输入"=w53) -> ("错误输出"=w50:errorcluster)
  n151 = call <vilib>:"Simple Error Handler.vi"("error in (no error)"=w1) -> ()  [unwired: 4 in, 5 out]
  n152 = call <vilib>:"Simple Error Handler.vi"() -> ()  [unwired: 5 in, 5 out]
  n153 = call <vilib>:"Simple Error Handler.vi"("error in (no error)"=w50) -> ()  [unwired: 4 in, 5 out]
  n154 = call <vilib>:"DAQmx Clear Task.vi"("task in"=w8) -> ()  [unwired: 14 in, 1 out]
  n155 = call <vilib>:"DAQmx Clear Task.vi"("task in"=w9) -> ()  [unwired: 14 in, 1 out]
